vi "Autonomous Independent.vi"() -> ()   [LabVIEW 2011]
doc: "This VI is called when autonomous begins, and will automatically be terminated when autonomous ends. You can carry out timed or sensor driven robot movement independently without needing to return to the caller."
uses:
  Robot Global Data.vi
  <vilib>/Rock Robotics/WPI/RobotDrive/WPI_RobotDriveArcadeDrive_Standard(NoSaturation).vi
panel:
  in  "offset":dbl=1.7
  in  "autonomous shot delay":dbl=0.5
  in  "autonomous speedScaling":dbl=0.39
  in  "autonomous axis 3 (throttle)":dbl=0.8
  in  "autonomous speedFactor":dbl=1.05
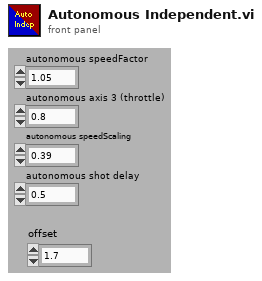
[diagram p1: front panel]
types:
  T1 = typedef "WPI_JoystickDevRef.ctl" = cluster{"Device":T2}
  T2 = typedef "WPI_JoystickDeviceEnum.ctl" = enum16{"USB 1", "USB 2", "USB 3", "USB 4", "Kinect 1", "Kinect 2"}
  T3 = cluster{"axis 1 (x)":dbl, "axis 2 (y)":dbl, "axis 3 (throttle)":dbl, "axis 4":dbl, "axis 5":dbl, "axis 6":dbl}
  T4 = typedef "WPI_RobotDriveDevRef.ctl" = cluster{"DevStatus":errorcluster, "Motors[]":T5[], "Square Inputs":bool, "Max Output":dbl, "Isochronous":bool}
  T5 = typedef "WPI_MotorControlDeviceRef.ctl" = cluster{"DeviceStatus":errorcluster, "Type":enum16{"PWM", "CAN"}, "PWM":cluster{"Digital Module":T6, "PWM Channel":T7, "DeadBand":T8}, "CAN":cluster{"Device Number":u8, "Control Mode":T9, "Semaphore":T10, "Max Vout":dbl}, "Invert":bool, "TransformRef":T11, "InvTransformRef":T11}
  T6 = typedef "FPGA_TypedefDigitalModule.ctl" = enum16{"Digital Module 1", "Digital Module 2"}
  T7 = typedef "FPGA_DIOPWMChannel.ctl" = enum8{"PWM 1", "PWM 2", "PWM 3", "PWM 4", "PWM 5", "PWM 6", "PWM 7", "PWM 8", "PWM 9", "PWM 10", "Invalid"}
  T8 = typedef "WPI_PWMDeadband.ctl" = cluster{"Name":string, "maxPositivePwm":i32, "minPositivePwm":i32, "centerPwm":i32, "maxNegativePwm":i32, "minNegativePwm":i32, "angularRange":u16}
  T9 = typedef "WPI_CANJaguar_ControlMode.ctl" = enum8{"Percent VBus", "Current", "Speed", "Position", "Voltage"}
  T10 = typedef "Semaphore RefNum" = refnum<k1>
  T11 = typedef "WPI_PWMTransform_ConPane.ctl" = refnum<vi>
  T12 = typedef "SkeletonVertexTrackState.ctl" = enum32{"NotTracked", "Inferred", "Tracked"}
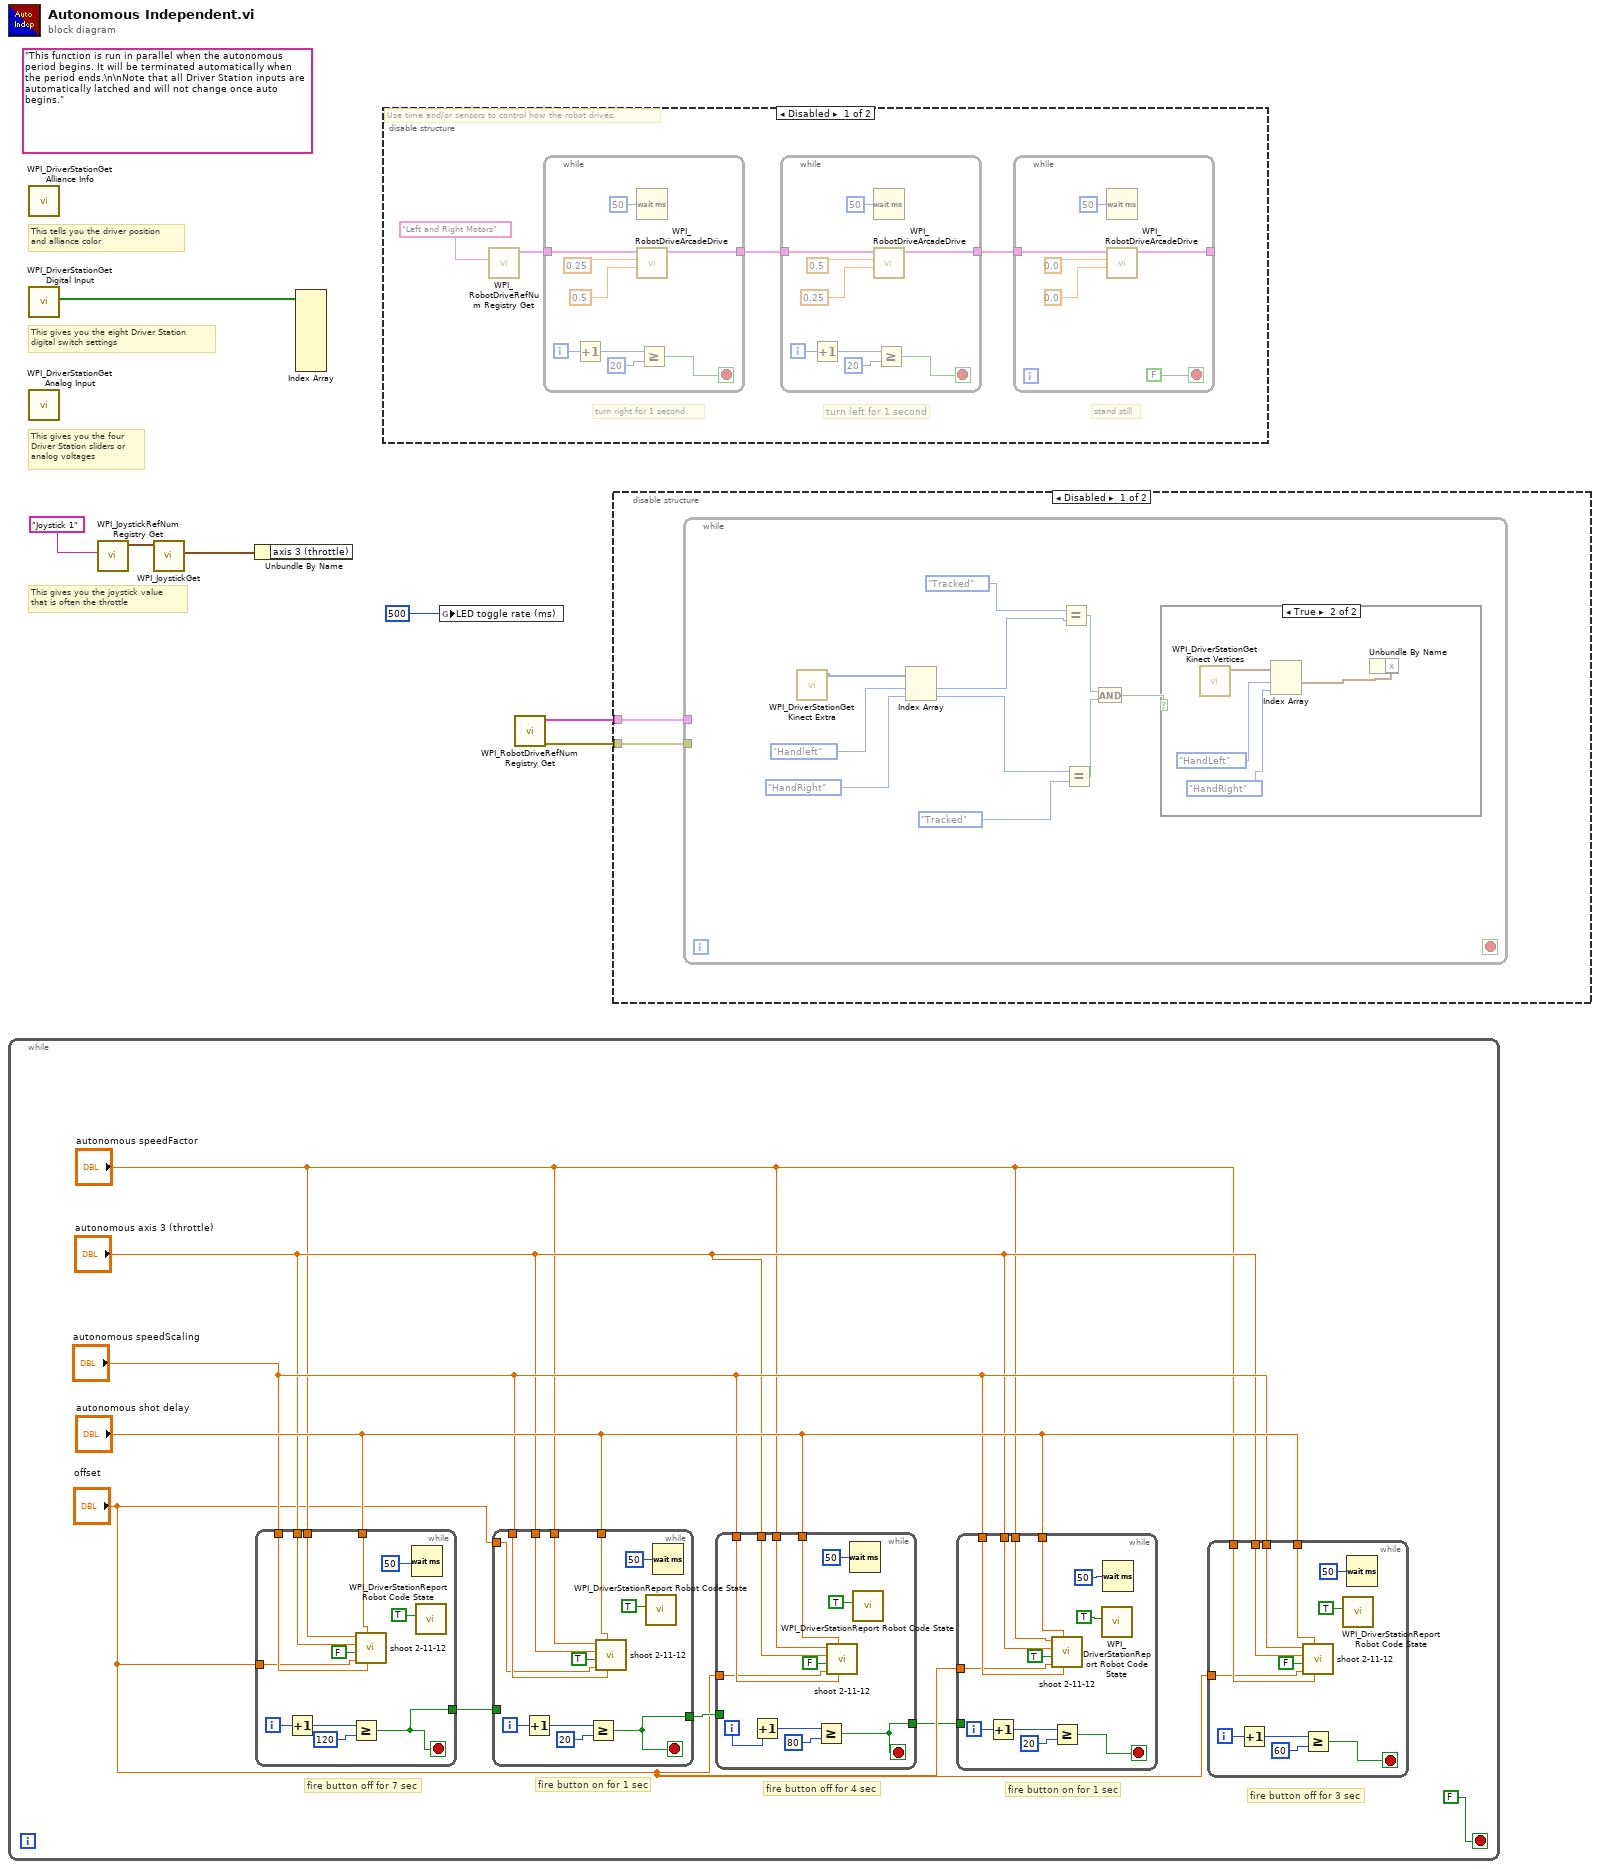
[diagram p0: block diagram]
diagram:
  (unwired) "This function is run in parallel when the autonomous period begins. It will be terminated automatically when the period ends.\n\nNote that all Driver Station inputs are automatically latched and will not change once auto begins."
  # "This gives you the joystick value\nthat is often the throttle"
  # "This tells you the driver position\nand alliance color"
  # "This gives you the eight Driver Station\ndigital switch settings"
  # "This gives you the four\nDriver Station sliders or\nanalog voltages"
  n1 = while {
    stop <- FALSE stop-if-true
    # "fire button off for 3 sec"
    # "fire button on for 1 sec"
    # "fire button off for 4 sec"
    # "fire button on for 1 sec"
    # "fire button off for 7 sec"
    n2 = while {
      tunnel: "autonomous speedFactor" -> [w72]
      tunnel: "autonomous axis 3 (throttle)" -> [w71]
      tunnel: "autonomous speedScaling" -> [w70]
      tunnel: "autonomous shot delay" -> [w69]
      tunnel: [w68] -> w16
      tunnel: "offset" -> [w66]
      i -> [w75]
      stop <- w68 stop-if-true
      n3 = Increment(x=w75) -> (x+1=w73:i32)
      n4 = Greater Or Equal?(x=w73, y=120) -> (x >= y?=w68:bool)
      n5 = call "shoot 2-11-12.vi"("speedScaling"=w70, "shot delay"=w69, "offset"=w66, "Button 1"=FALSE, "axis 3 (throttle)"=w71, "speedFactor"=w72) -> ()  [unwired: 6 in]
      n6 = Wait (ms)(milliseconds to wait=u32 50) -> ()  [unwired: 1 out]
      n7 = call <vilib>:"WPI_DriverStationReport Robot Code State.vi"("Autonomous"=TRUE) -> ()  [unwired: 10 in, 1 out]
    }
    n8 = while {
      tunnel: "autonomous speedFactor" -> [w60]
      tunnel: "autonomous axis 3 (throttle)" -> [w59]
      tunnel: "autonomous speedScaling" -> [w58]
      tunnel: "autonomous shot delay" -> [w57]
      tunnel: w16 -> [_]
      tunnel: [w55] -> w15
      tunnel: "offset" -> [w54]
      i -> [w63]
      stop <- w55 stop-if-true
      n9 = Increment(x=w63) -> (x+1=w61:i32)
      n10 = Greater Or Equal?(x=w61, y=20) -> (x >= y?=w55:bool)
      n11 = call "shoot 2-11-12.vi"("speedScaling"=w58, "shot delay"=w57, "offset"=w54, "Button 1"=TRUE, "axis 3 (throttle)"=w59, "speedFactor"=w60) -> ()  [unwired: 6 in]
      n12 = call <vilib>:"WPI_DriverStationReport Robot Code State.vi"("Autonomous"=TRUE) -> ()  [unwired: 10 in, 1 out]
      n13 = Wait (ms)(milliseconds to wait=u32 50) -> ()  [unwired: 1 out]
    }
    n14 = while {
      tunnel: "autonomous speedFactor" -> [w51]
      tunnel: "autonomous axis 3 (throttle)" -> [w50]
      tunnel: "autonomous speedScaling" -> [w49]
      tunnel: "autonomous shot delay" -> [w48]
      tunnel: w15 -> [_]
      tunnel: [w43] -> w8
      tunnel: "offset" -> [w42]
      i -> [w44]
      stop <- w43 stop-if-true
      n15 = Increment(x=w44) -> (x+1=w45:i32)
      n16 = Greater Or Equal?(x=w45, y=80) -> (x >= y?=w43:bool)
      n17 = call "shoot 2-11-12.vi"("speedScaling"=w49, "shot delay"=w48, "offset"=w42, "Button 1"=FALSE, "axis 3 (throttle)"=w50, "speedFactor"=w51) -> ()  [unwired: 6 in]
      n18 = Wait (ms)(milliseconds to wait=u32 50) -> ()  [unwired: 1 out]
      n19 = call <vilib>:"WPI_DriverStationReport Robot Code State.vi"("Autonomous"=TRUE) -> ()  [unwired: 10 in, 1 out]
    }
    n20 = while {
      tunnel: "autonomous speedFactor" -> [w35]
      tunnel: "autonomous axis 3 (throttle)" -> [w34]
      tunnel: "autonomous speedScaling" -> [w33]
      tunnel: "autonomous shot delay" -> [w32]
      tunnel: w8 -> [_]
      tunnel: "offset" -> [w30]
      i -> [w39]
      stop <- w37 stop-if-true
      n21 = Increment(x=w39) -> (x+1=w36:i32)
      n22 = call "shoot 2-11-12.vi"("speedScaling"=w33, "shot delay"=w32, "offset"=w30, "Button 1"=TRUE, "axis 3 (throttle)"=w34, "speedFactor"=w35) -> ()  [unwired: 6 in]
      n23 = Greater Or Equal?(x=w36, y=20) -> (x >= y?=w37:bool)
      n24 = call <vilib>:"WPI_DriverStationReport Robot Code State.vi"("Autonomous"=TRUE) -> ()  [unwired: 10 in, 1 out]
      n25 = Wait (ms)(milliseconds to wait=u32 50) -> ()  [unwired: 1 out]
    }
    n26 = while {
      tunnel: "autonomous speedScaling" -> [w23]
      tunnel: "autonomous axis 3 (throttle)" -> [w22]
      tunnel: "autonomous speedFactor" -> [w21]
      tunnel: "autonomous shot delay" -> [w20]
      tunnel: "offset" -> [w18]
      i -> [w27]
      stop <- w25 stop-if-true
      n27 = Increment(x=w27) -> (x+1=w24:i32)
      n28 = call "shoot 2-11-12.vi"("speedScaling"=w21, "shot delay"=w20, "offset"=w18, "Button 1"=FALSE, "axis 3 (throttle)"=w22, "speedFactor"=w23) -> ()  [unwired: 6 in]
      n29 = Greater Or Equal?(x=w24, y=60) -> (x >= y?=w25:bool)
      n30 = call <vilib>:"WPI_DriverStationReport Robot Code State.vi"("Autonomous"=TRUE) -> ()  [unwired: 10 in, 1 out]
      n31 = Wait (ms)(milliseconds to wait=u32 50) -> ()  [unwired: 1 out]
    }
  }
  n32 = call <vilib>:"WPI_DriverStationGet Alliance Info.vi"() -> ()  [unwired: 12 out]
  n33 = call <vilib>:"WPI_DriverStationGet Digital Input.vi"() -> ("Driver Station Digital Input (1-8)"=w7:bool[])  [unwired: 11 out]
  n34 = call <vilib>:"WPI_DriverStationGet Analog Input.vi"() -> ()  [unwired: 12 out]
  n35 = call <vilib>:"WPI_JoystickRefNum Registry Get.vi"("refnum name"="Joystick 1") -> ("JoystickDevRef"=w4:T1)  [unwired: 1 in, 9 out]
  n36 = call <vilib>:"WPI_JoystickGet.vi"("JoystickDevRef"=w4) -> ("Axes"=w5:T3)  [unwired: 1 in, 5 out]
  n37 = Unbundle By Name(w5) -> ()  [unwired: 1 out]
  n38 = Index Array(array=w7) -> ()  [unwired: 8 in, 8 out]
  n39 = disable-structure shown="Disabled" {
    frame Disabled {
      # "stand still"
      # "turn left for 1 second"
      # "turn right for 1 second"
      # "Use time and/or sensors to control how the robot drives."
      n40 = call <vilib>:"WPI_RobotDriveRefNum Registry Get.vi"("refnum name"="Left and Right Motors") -> ("RobotDriveDevRef"=w79:T4)  [unwired: 1 in, 9 out]
      n41 = while {
        tunnel: w79 -> [w104]
        tunnel: [w97] -> w78
        i -> [w100]
        stop <- w98 stop-if-true
        n42 = Increment(x=w100) -> (x+1=w96:i32)
        n43 = Wait (ms)(milliseconds to wait=u32 50) -> ()  [unwired: 1 out]
        n44 = call-poly <vilib>:"WPI_RobotDriveArcadeDrive.vi"("Y axis value"=0.5 ("X axis value"), "X axis value"=0.25, "RobotDriveDevRef"=w104) -> ("RobotDriveDevRef"=w97:T4)  [unwired: 1 in, 7 out]
        n45 = Greater Or Equal?(x=w96, y=20) -> (x >= y?=w98:bool)
      }
      n46 = while {
        tunnel: w78 -> [w95]
        tunnel: [w88] -> w77
        i -> [w91]
        stop <- w89 stop-if-true
        n47 = Increment(x=w91) -> (x+1=w87:i32)
        n48 = Wait (ms)(milliseconds to wait=u32 50) -> ()  [unwired: 1 out]
        n49 = call-poly <vilib>:"WPI_RobotDriveArcadeDrive.vi"("Y axis value"=0.25 ("X axis value"), "X axis value"=0.5, "RobotDriveDevRef"=w95) -> ("RobotDriveDevRef"=w88:T4)  [unwired: 1 in, 7 out]
        n50 = Greater Or Equal?(x=w87, y=20) -> (x >= y?=w89:bool)
      }
      n51 = while {
        tunnel: w77 -> [w86]
        tunnel: [w82] -> _
        stop <- FALSE stop-if-true
        n52 = Wait (ms)(milliseconds to wait=u32 50) -> ()  [unwired: 1 out]
        n53 = call-poly <vilib>:"WPI_RobotDriveArcadeDrive.vi"("Y axis value"=0.0 ("X axis value"), "X axis value"=0.0, "RobotDriveDevRef"=w86) -> ("RobotDriveDevRef"=w82:T4)  [unwired: 1 in, 7 out]
      }
    }
    frame Enabled {
    }
  }
  n54 = global write "Robot Global Data.vi" "LED toggle rate (ms)"(u32 500 ("LED ms toggle rate")) -> ()
  n55 = call <vilib>:"WPI_RobotDriveRefNum Registry Get.vi"() -> ("error out"=w2:errorcluster, "RobotDriveDevRef"=w1:T4)  [unwired: 10 in]
  n56 = disable-structure shown="Disabled" {
    disable-tunnel: w2 -> [w106 _]
    disable-tunnel: w1 -> [w105 _]
    frame Disabled {
      n57 = while {
        tunnel: w106 -> [_]
        tunnel: w105 -> [_]
        stop <- _ stop-if-true
        n58 = call <vilib>:"WPI_DriverStationGet Kinect Extra.vi"() -> ("Skeleton Tracking State"=w116:T12[])  [unwired: 7 in, 4 out]
        n59 = Index Array(array=w116, index #1=enum16{"Handleft"}."Handleft", index #2=enum16{"HandRight"}."HandRight") -> (element #1=w112:T12, element #2=w113:T12)
        n60 = Equal?(x=enum16{"Tracked"}."Tracked", y=w112) -> (x = y?=w108:bool)
        n61 = Equal?(x=w113, y=enum16{"Tracked"}."Tracked") -> (x = y?=w109:bool)
        n62 = And(x=w108, y=w109) -> (x .and. y?=w107:bool)
        n63 = case shown="True" w107 {
          frame False {
          }
          frame True {
            n64 = call <vilib>:"WPI_DriverStationGet Kinect Vertices.vi"() -> ("Skeleton Vertices"=w120:cluster{"x":sgl, "y":sgl, "z":sgl}[])  [unwired: 10 in, 1 out]
            n65 = Index Array(array=w120, index #1=enum16{"HandLeft"}."HandLeft", index #2=enum16{"HandRight"}."HandRight") -> (element #1=w117:cluster{"x":sgl, "y":sgl, "z":sgl})  [unwired: 1 out]
            n66 = Unbundle By Name(w117) -> ()  [unwired: 1 out]
          }
        }
      }
    }
    frame Enabled {
    }
  }
